vi "FormulaValues.vi"(2 "X End":dbl, 3 "X Start":dbl, 4 "b":dbl, 5 "k":dbl) -> (0 "YEnd":dbl, 1 "YStart":dbl)   [LabVIEW 2011]
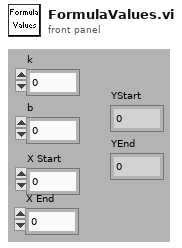
[diagram p1: front panel]
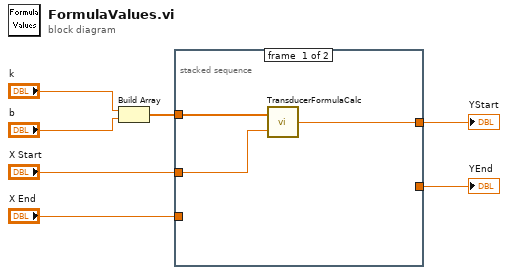
[diagram p0: block diagram]
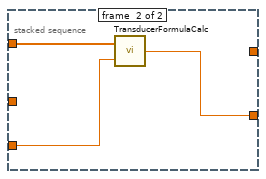
[diagram p2: hidden frame]
diagram:
  n1 = Build Array("k", "b") -> (w1:dbl[])
  n2 = stacked-sequence {
    tunnel: "X Start" -> [w10 _]
    tunnel: "X End" -> [_ w13]
    tunnel: [w9 _] -> w5
    tunnel: [_ w12] -> w4
    tunnel: w1 -> [w8 w11]
    frame #0 {
      n3 = call "TransducerFormulaCalc.vi"("X"=w10, "公式参数"=w8) -> ("Y"=w9:dbl)
    }
    frame #1 {
      n4 = call "TransducerFormulaCalc.vi"("X"=w13, "公式参数"=w11) -> ("Y"=w12:dbl)
    }
  }
  "YStart" <- w5
  "YEnd" <- w4
